vi "Fix CLFN Paths.vi"() -> ()   [LabVIEW 2019]
uses:
  <vilib>/Utility/traverseref.llb/TRef TravTarget.ctl
  <vilib>/Utility/traverseref.llb/VI Scripting - Traverse.lvlib
panel:
  out "Checking/Updating...":path
  # "This VI will walk the grpc-support.lvlib for .vi and .vim files\n\nAny Call Library Function nodes in those vis/vims will be checked.\n\nCLFNs with the \"Specify Path on Diagram\", the path will be cleared otherwise the path will be set \nto the the name of the resource directory for this LV Version with a library name of labview_grpc_server.*"
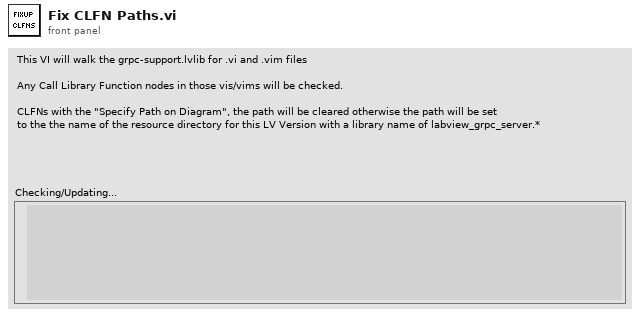
[diagram p1: front panel]
types:
  T1 = typedef "TRef TravTarget.ctl" = enum16{"FP", "BD", "Other"}
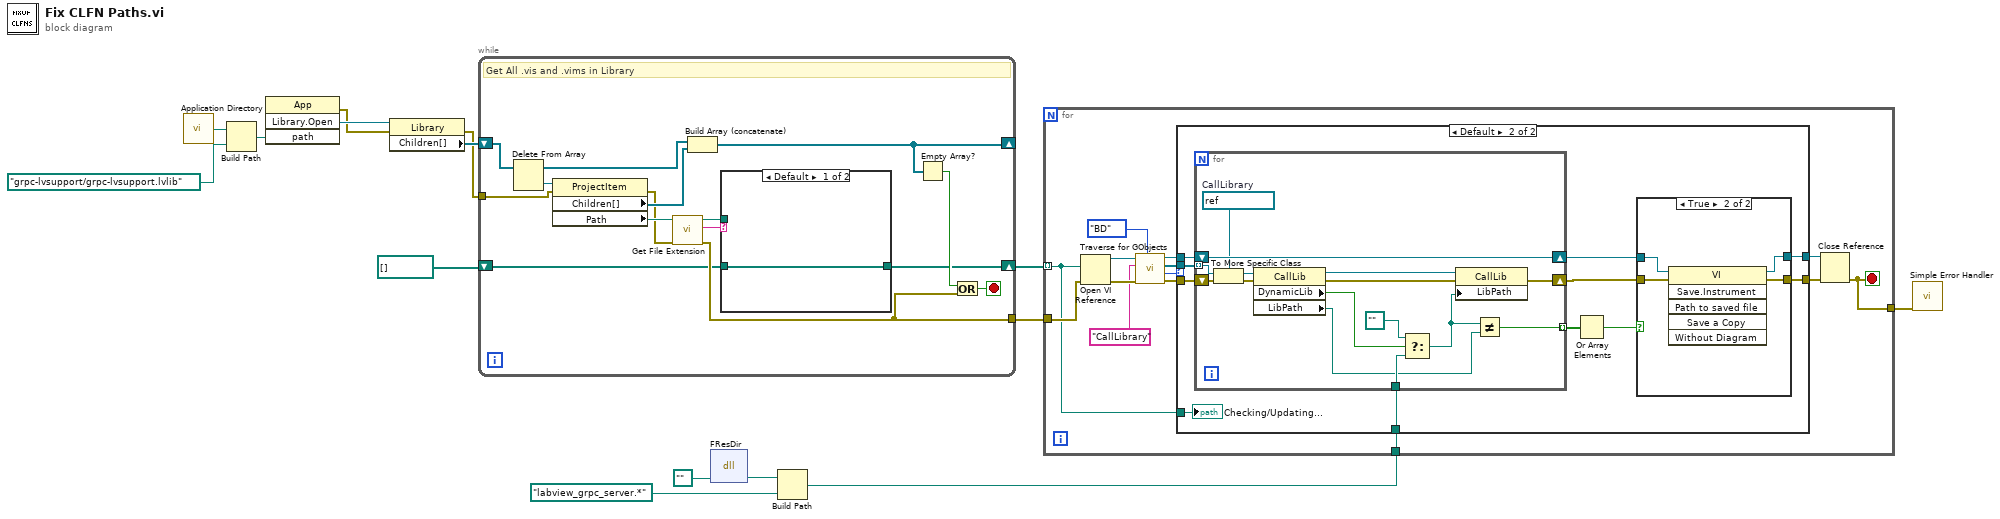
[diagram p0: block diagram]
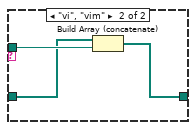
[diagram p4: hidden frame]
diagram:
  n1 = call <vilib>:"Application Directory.vi"() -> ("Application Directory"=w15:path)
  n2 = Build Path(base path=w15, name or relative path=path "grpc-lvsupport/grpc-lvsupport.lvlib") -> (appended path=w13:path)
  n3 = invoke class="App" method="Library.Open"("path"=w13) -> (error out=w10:errorcluster, "Open Library"=w12:refnum<vi>)  [unwired: 3 in, 2 out]
  n4 = property class="Library"(reference=w12, error in=w10) -> (error out=w9:errorcluster, "Children[]"=w11:refnum<vi>[])  [unwired: 1 out]
  n5 = while {
    shift-right: [w26] -> _
    shift-left: w11 -> [w30]
    tunnel: w9 -> [w21]
    tunnel: [w18] -> w6
    shift-right: [w16] -> w7
    shift-left: path[] [] ("appended array") -> [w17]
    stop <- w19 stop-if-true
    # "Get All .vis and .vims in Library"
    n6 = Delete From Array(array=w30) -> (deleted portion=w29:refnum<vi>, array with subset deleted=w28:refnum<vi>[])  [unwired: 2 in]
    n7 = property class="ProjectItem"(reference=w29, error in=w21) -> (error out=w20:errorcluster, "Children[]"=w27:refnum<vi>[], "Path"=w24:path)  [unwired: 1 out]
    n8 = call <vilib>:"Get File Extension.vi"("error in (no error)"=w20, "file"=w24) -> ("error out"=w18:errorcluster, "lowercase file extension"=w23:string, "dup file"=w22:path)  [unwired: 5 in, 2 out]
    n9 = Build Array (concatenate)(w28, w27) -> (w26:refnum<vi>[])
    n10 = case shown="Default" w23 {
      tunnel: w22 -> [_ w34]
      tunnel: w17 -> [w31 w33]
      tunnel: [w31 w32] -> w16
      frame Default {
      }
      frame "vi", "vim" {
        n11 = Build Array (concatenate)(w33, w34) -> (w32:path[])
      }
    }
    n12 = Empty Array?(array=w26) -> (empty?=w25:bool)
    n13 = Or(x=w25, y=w18) -> (x .or. y?=w19:bool)
  }
  n14 = dll-call lib="LabVIEW" fn="FResDir"("Path"=path "") -> ("Path"=w4:path)  [unwired: 4 in, 2 out]
  n15 = Build Path(base path=w4, name or relative path=path "labview_grpc_server.*" ("Path")) -> (appended path=w2:path)
  n16 = for {
    tunnel: w7 -> [w36] mode=indexing
    tunnel: w6 -> [w48]
    tunnel: w2 -> [w41]
    tunnel: [w35] -> w1
    stop <- w35 stop-if-true
    n17 = Open VI Reference(vi path=w36, error in (no error)=w48) -> (vi reference=w47:refnum<vi>, error out=w46:errorcluster)  [unwired: 4 in]
    n18 = call <vilib>:"Traverse for GObjects.vi"("Traverse Target"=TRef_TravTarget."BD", "error in (no error)"=w46, "Class Name"="CallLibrary", "VI Refnum"=w47) -> ("error out"=w43:errorcluster, "# of Refs"=w39:i32, "References"=w44:refnum<vi>[], "dup VI Refnum"=w40:refnum<vi>)  [unwired: 4 in]
    n19 = case shown="Default" w39 {
      tunnel: w44 -> [_ w61]
      tunnel: w43 -> [w49 w60]
      tunnel: w41 -> [_ w59]
      tunnel: w40 -> [w50 w58]
      tunnel: [w50 w55] -> w37
      tunnel: [w49 w54] -> w38
      tunnel: w36 -> [_ w51]
      frame ..0 {
      }
      frame Default {
        n20 = for {
          tunnel: w61 -> [w82] mode=indexing
          tunnel: w59 -> [w74]
          shift-right: [w72] -> w57
          shift-left: w58 -> [w72]
          shift-right: [w73] -> w56
          shift-left: w60 -> [w81]
          tunnel: [w68] -> w53 mode=indexing
          w71 = refnum<vi> refnum  # CallLibrary
          n21 = To More Specific Class(target class=w71, reference=w82, error in=w81) -> (specific class reference=w79:refnum<vi>, error out=w80:errorcluster)
          n22 = property class="CallLib"(reference=w79, error in=w80) -> (reference out=w78:refnum<vi>, error out=w77:errorcluster, "DynamicLib"=w76:bool, "LibPath"=w69:path)
          n23 = Select(t=path "", s=w76, f=w74) -> (s? t:f=w70:path)
          n24 = property class="CallLib"(reference=w78, error in=w77, "LibPath"=w70) -> (error out=w73:errorcluster)  [unwired: 1 out]
          n25 = Not Equal?(x=w70, y=w69) -> (x != y?=w68:bool)
        }
        n26 = Or Array Elements(Boolean array=w53) -> (logical OR=w52:bool)
        n27 = case shown="True" w52 {
          tunnel: w57 -> [w63 w67]
          tunnel: w56 -> [w62 w66]
          tunnel: [w63 w65] -> w55
          tunnel: [w62 w64] -> w54
          frame False {
          }
          frame True {
            n28 = invoke class="VI" method="Save.Instrument"(reference=w67, error in=w66) -> (reference out=w65:refnum<vi>, error out=w64:errorcluster)  [unwired: 4 in, 4 out]
          }
        }
        "Checking/Updating..." <- w51
      }
    }
    n29 = Close Reference(reference=w37, error in (no error)=w38) -> (error out=w35:errorcluster)
  }
  n30 = call <vilib>:"Simple Error Handler.vi"("error in (no error)"=w1) -> ()  [unwired: 4 in, 5 out]
